vi "InitDrive.vi"   [LabVIEW 2019]
doc: "This VI initializes devices related directly to the drive subsystem."
uses:
  <vilib>/Rock Robotics/WPI/Solenoid/WPI_SolenoidChannel.ctl
  <vilib>/Rock Robotics/WPI/ThirdParty/Phoenix-LabVIEW/Motor Controller/Controls/CTRE_Phoenix_MotorControl_NeutralMode.ctl
  <vilib>/Rock Robotics/WPI/ThirdParty/Phoenix-LabVIEW/Motor Controller/Controls/CTRE_Phoenix_MotorControl_SupplyCurrentLimitConfiguration.ctl
  <vilib>/Rock Robotics/WPI/ThirdParty/Phoenix-LabVIEW/Motor Controller/Controls/CTRE_Phoenix_MotorControl_TalonFXInvertType.ctl
  <vilib>/Rock Robotics/WPI/ThirdParty/Phoenix-LabVIEW/Motor Controller/Controls/CTRE_Phoenix_MotorControl_FeedbackDevice_TalonFX.ctl
  <vilib>/Rock Robotics/WPI/Solenoid/WPI_SolenoidOpenDouble.vi
  refnums.vi
types:
  T1 = typedef "WPI_SolenoidChannel.ctl" = enum8{"Solenoid 0", "Solenoid 1", "Solenoid 2", "Solenoid 3", "Solenoid 4", "Solenoid 5", "Solenoid 6", "Solenoid 7", "Invalid"}
  T2 = typedef "CTRE_Phoenix_MotorControl_TalonFXInvertType.ctl" = enum16{"Counter-Clockwise", "Clockwise"}
  T3 = typedef "CTRE_Phoenix_MotorControl_FeedbackDevice_TalonFX.ctl" = i8
  T4 = typedef "CTRE_Phoenix_MotorControl_SupplyCurrentLimitConfiguration.ctl" = cluster{"Enable?":bool, "Current Limit":dbl, "Threshold Current":dbl, "Threshold Time":dbl}
  T5 = typedef "CTRE_Phoenix_MotorControl_NeutralMode.ctl" = enum8{"EEPROMSetting", "Override to Coast", "Override to Brake"}
  T6 = typedef "WPI_MotorControlDeviceRef.ctl" = cluster{"DeviceStatus":errorcluster, "Type":T7, "PWM":cluster{"PWM Channel":T8, "DeadBand":T9}, "CAN":cluster{"Device Number":u8, "SetOutput VI Ref":variant, "GetOutput VI Ref":variant, "Enable VI Ref":variant, "Disable VI Ref":variant, "Data":variant}, "Invert":bool, "DIO PWM":cluster{"PWM \"Enable\" Channel":T8, "DIOChannel":T10, "PWM Rate":dbl}}
  T7 = typedef "WPI_MotorControlType.ctl" = enum16{"PWM", "CAN", "DIO PWM"}
  T8 = typedef "FPGA_DIOPWMChannel.ctl" = enum8{"PWM 0", "PWM 1", "PWM 2", "PWM 3", "PWM 4", "PWM 5", "PWM 6", "PWM 7", "PWM 8", "PWM 9", "PWM MXP 0", "PWM MXP 1", "PWM MXP 2", "PWM MXP 3", "PWM MXP 4", "PWM MXP 5", "PWM MXP 6", "PWM MXP 7", "PWM MXP 8", "PWM MXP 9", "Invalid"}
  T9 = typedef "WPI_PWMDeadband.ctl" = cluster{"Name":string, "maxPositivePwm":i32, "minPositivePwm":i32, "centerPwm":i32, "maxNegativePwm":i32, "minNegativePwm":i32, "angularRange":u16}
  T10 = typedef "FPGA_DIOChannel.ctl" = enum8{"DIO 0", "DIO 1", "DIO 2", "DIO 3", "DIO 4", "DIO 5", "DIO 6", "DIO 7", "DIO 8", "DIO 9", "DIO MXP 0", "DIO MXP 1", "DIO MXP 2", "DIO MXP 3", "DIO MXP 4", "DIO MXP 5", "DIO MXP 6", "DIO MXP 7", "DIO MXP 8", "DIO MXP 9", "DIO MXP 10", "DIO MXP 11", "DIO MXP 12", "DIO MXP 13", "DIO MXP 14", "DIO MXP 15", "SPI Port CS1", "SPI Port CS2", "SPI Port CS3", "SPI Port MISO", "SPI Port MOSI", "Invalid"}
  T11 = typedef "WPI_SolenoidDevRef.ctl" = cluster{"DevStatus":errorcluster, "Pneumatics Control Module":u8, "Forward Solenoid Channel":T1, "Reverse Solenoid Channel":T1}
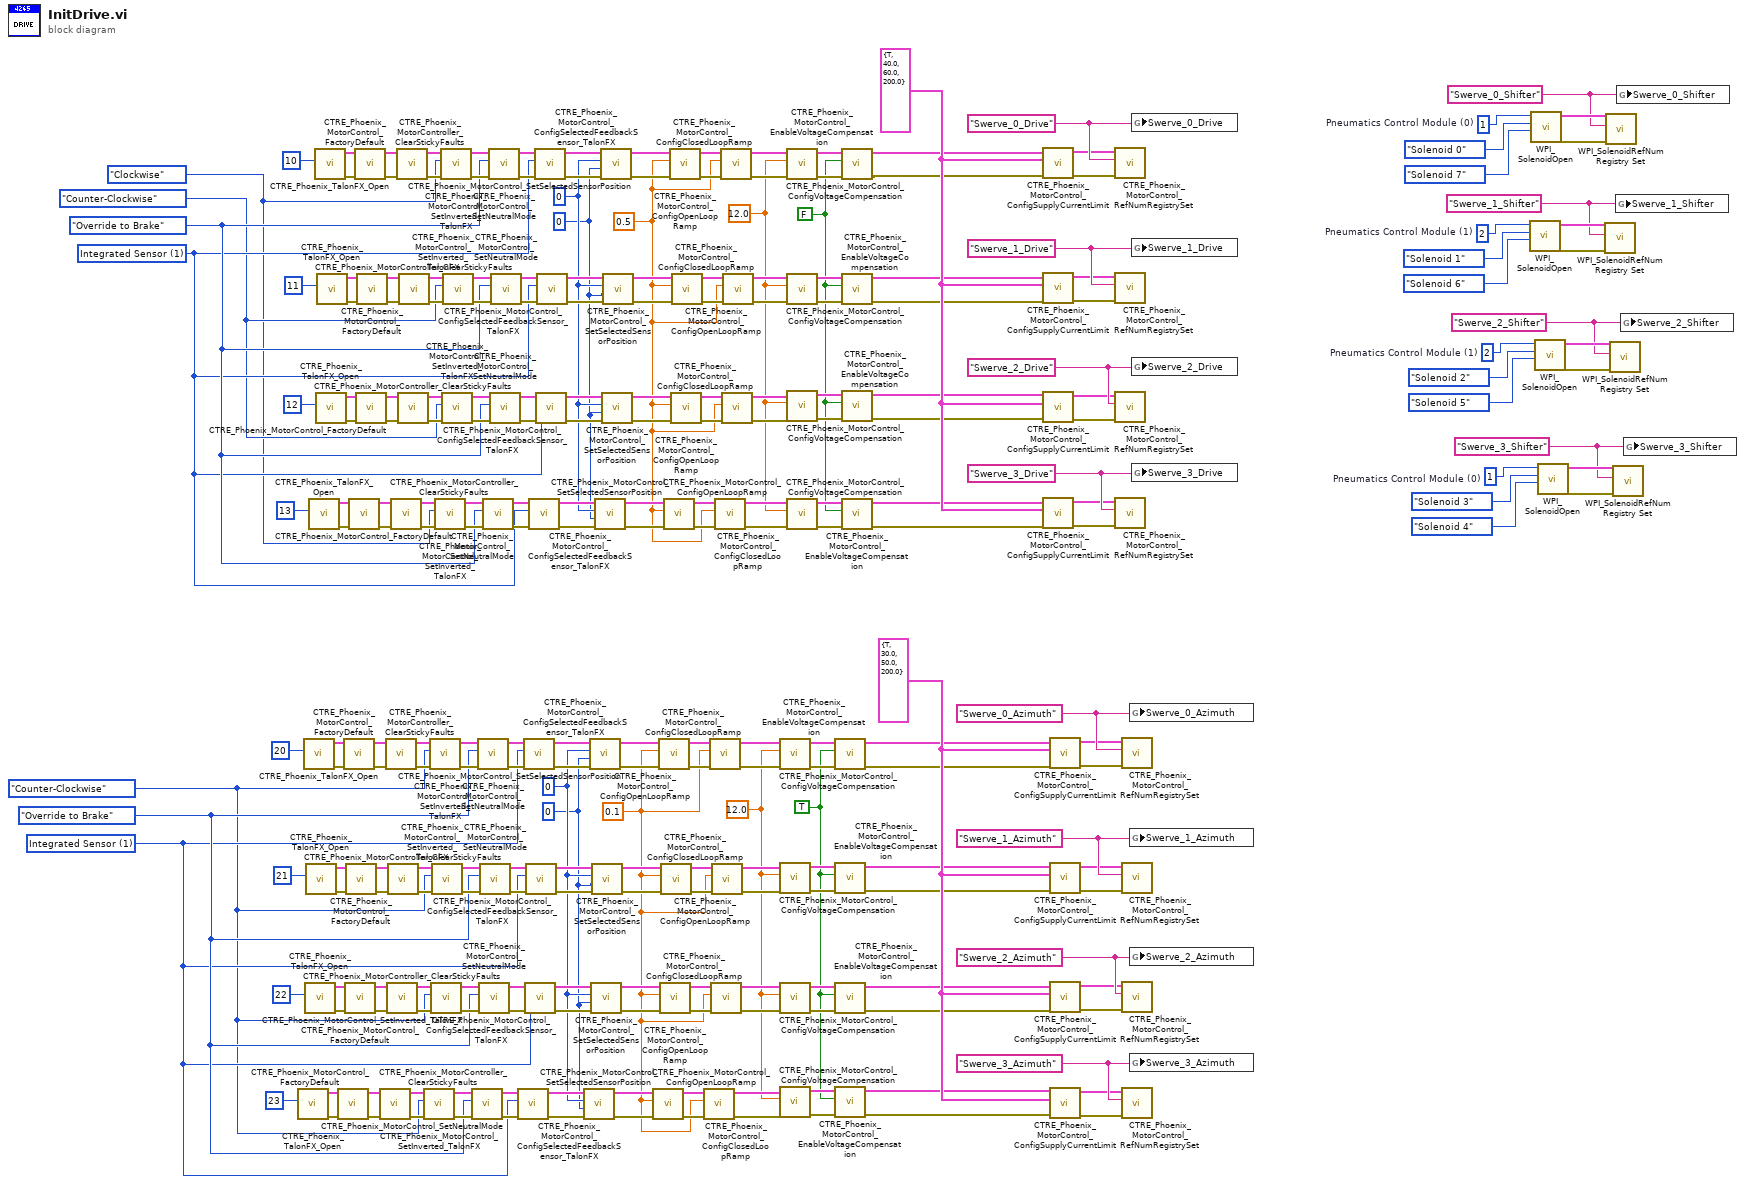
[diagram p0: block diagram]
diagram:
  w2 = "Swerve_0_Shifter" ("refnum name")
  w7 = u8 1  # Pneumatics Control Module (0)
  w8 = "Swerve_1_Shifter" ("refnum name")
  w13 = u8 2  # Pneumatics Control Module (1)
  w14 = "Swerve_2_Shifter" ("refnum name")
  w19 = u8 2  # Pneumatics Control Module (1)
  w22 = CTRE_Phoenix_MotorControl_TalonFXInvertType."Clockwise" ("Invert Type")
  w24 = TRUE ("Enable Voltage Compensation?")
  w25 = 12.0 ("Saturation Voltage")
  w26 = FALSE ("Enable Voltage Compensation?")
  w27 = 12.0 ("Saturation Voltage")
  w74 = T3 1 items=["Integrated Sensor"=1, "Sensor Sum (S0 + S1)"=9, "Sensor Difference (D0 - D1)"=10, "Remote Source 0"=11, "Remote Source 1"=12, "None"=14, "Software Emulated"=15] ("Talon FX Feedback Device")
  w79 = T4 {"Enable?"=TRUE, "Current Limit"=30.0, "Threshold Current"=50.0, "Threshold Time"=200.0} ("Supply Current Limit Configuration")
  w75 = 0.1 ("secondsFromNeutralToFull")
  w76 = u32 0 ("pidLoopIdx")
  w77 = 0 ("New Sensor Position")
  w78 = CTRE_Phoenix_MotorControl_NeutralMode."Override to Brake" ("Motor Control Neutral Mode")
  w1 = CTRE_Phoenix_MotorControl_TalonFXInvertType."Counter-Clockwise" ("Invert Type")
  w95 = "Swerve_0_Azimuth" ("refnum name")
  w115 = "Swerve_1_Azimuth" ("refnum name")
  w135 = "Swerve_2_Azimuth" ("refnum name")
  w155 = "Swerve_3_Azimuth" ("refnum name")
  w163 = T3 1 items=["Integrated Sensor"=1, "Sensor Sum (S0 + S1)"=9, "Sensor Difference (D0 - D1)"=10, "Remote Source 0"=11, "Remote Source 1"=12, "None"=14, "Software Emulated"=15] ("Talon FX Feedback Device")
  w165 = T4 {"Enable?"=TRUE, "Current Limit"=40.0, "Threshold Current"=60.0, "Threshold Time"=200.0} ("Supply Current Limit Configuration")
  w160 = 0.5 ("secondsFromNeutralToFull")
  w161 = u32 0 ("pidLoopIdx")
  w162 = 0 ("New Sensor Position")
  w164 = CTRE_Phoenix_MotorControl_NeutralMode."Override to Brake" ("Motor Control Neutral Mode")
  w23 = CTRE_Phoenix_MotorControl_TalonFXInvertType."Counter-Clockwise" ("Invert Type")
  w181 = "Swerve_0_Drive" ("refnum name")
  w201 = "Swerve_1_Drive" ("refnum name")
  w221 = "Swerve_2_Drive" ("refnum name")
  w241 = "Swerve_3_Drive" ("refnum name")
  w246 = "Swerve_3_Shifter" ("refnum name")
  w251 = u8 1  # Pneumatics Control Module (0)
  n1 = call <vilib>:"CTRE_Phoenix_TalonFX_Open.vi"("Device Number"=u8 23 ("Drive 4L")) -> ("error out"=w144:errorcluster, "CAN Talon SRX Ref"=w151:T6)  [unwired: 9 in]
  n2 = call <vilib>:"CTRE_Phoenix_TalonFX_Open.vi"("Device Number"=u8 20 ("Drive 4L")) -> ("error out"=w84:errorcluster, "CAN Talon SRX Ref"=w91:T6)  [unwired: 9 in]
  n3 = call <vilib>:"CTRE_Phoenix_TalonFX_Open.vi"("Device Number"=u8 22 ("Drive 4L")) -> ("error out"=w124:errorcluster, "CAN Talon SRX Ref"=w131:T6)  [unwired: 9 in]
  n4 = call <vilib>:"CTRE_Phoenix_TalonFX_Open.vi"("Device Number"=u8 21 ("Drive 4L")) -> ("error out"=w104:errorcluster, "CAN Talon SRX Ref"=w111:T6)  [unwired: 9 in]
  n5 = call <vilib>:"CTRE_Phoenix_TalonFX_Open.vi"("Device Number"=u8 13 ("Drive 4L")) -> ("error out"=w230:errorcluster, "CAN Talon SRX Ref"=w237:T6)  [unwired: 9 in]
  n6 = call <vilib>:"CTRE_Phoenix_TalonFX_Open.vi"("Device Number"=u8 10 ("Drive 4L")) -> ("error out"=w170:errorcluster, "CAN Talon SRX Ref"=w177:T6)  [unwired: 9 in]
  n7 = call <vilib>:"CTRE_Phoenix_TalonFX_Open.vi"("Device Number"=u8 12 ("Drive 4L")) -> ("error out"=w210:errorcluster, "CAN Talon SRX Ref"=w217:T6)  [unwired: 9 in]
  n8 = call <vilib>:"CTRE_Phoenix_TalonFX_Open.vi"("Device Number"=u8 11 ("Drive 4L")) -> ("error out"=w190:errorcluster, "CAN Talon SRX Ref"=w197:T6)  [unwired: 9 in]
  n9 = call <vilib>:"CTRE_Phoenix_MotorControl_FactoryDefault.vi"("error in"=w144, "PhoenixMotorControlDevRef"=w151) -> ("error out"=w147:errorcluster, "PhoenixMotorControlDevRef"=w148:T6)  [unwired: 8 in]
  n10 = call <vilib>:"CTRE_Phoenix_MotorControl_FactoryDefault.vi"("error in"=w84, "PhoenixMotorControlDevRef"=w91) -> ("error out"=w87:errorcluster, "PhoenixMotorControlDevRef"=w88:T6)  [unwired: 8 in]
  n11 = call <vilib>:"CTRE_Phoenix_MotorControl_FactoryDefault.vi"("error in"=w124, "PhoenixMotorControlDevRef"=w131) -> ("error out"=w127:errorcluster, "PhoenixMotorControlDevRef"=w128:T6)  [unwired: 8 in]
  n12 = call <vilib>:"CTRE_Phoenix_MotorControl_FactoryDefault.vi"("error in"=w104, "PhoenixMotorControlDevRef"=w111) -> ("error out"=w107:errorcluster, "PhoenixMotorControlDevRef"=w108:T6)  [unwired: 8 in]
  n13 = call <vilib>:"CTRE_Phoenix_MotorControl_FactoryDefault.vi"("error in"=w230, "PhoenixMotorControlDevRef"=w237) -> ("error out"=w233:errorcluster, "PhoenixMotorControlDevRef"=w234:T6)  [unwired: 8 in]
  n14 = call <vilib>:"CTRE_Phoenix_MotorControl_FactoryDefault.vi"("error in"=w170, "PhoenixMotorControlDevRef"=w177) -> ("error out"=w173:errorcluster, "PhoenixMotorControlDevRef"=w174:T6)  [unwired: 8 in]
  n15 = call <vilib>:"CTRE_Phoenix_MotorControl_FactoryDefault.vi"("error in"=w210, "PhoenixMotorControlDevRef"=w217) -> ("error out"=w213:errorcluster, "PhoenixMotorControlDevRef"=w214:T6)  [unwired: 8 in]
  n16 = call <vilib>:"CTRE_Phoenix_MotorControl_FactoryDefault.vi"("error in"=w190, "PhoenixMotorControlDevRef"=w197) -> ("error out"=w193:errorcluster, "PhoenixMotorControlDevRef"=w194:T6)  [unwired: 8 in]
  n17 = call <vilib>:"CTRE_Phoenix_MotorController_ClearStickyFaults.vi"("error in"=w147, "PhoenixMotorControlDevRef"=w148) -> ("error out"=w146:errorcluster, "PhoenixMotorControlDevRef"=w145:T6)  [unwired: 8 in]
  n18 = call <vilib>:"CTRE_Phoenix_MotorController_ClearStickyFaults.vi"("error in"=w87, "PhoenixMotorControlDevRef"=w88) -> ("error out"=w86:errorcluster, "PhoenixMotorControlDevRef"=w85:T6)  [unwired: 8 in]
  n19 = call <vilib>:"CTRE_Phoenix_MotorController_ClearStickyFaults.vi"("error in"=w127, "PhoenixMotorControlDevRef"=w128) -> ("error out"=w126:errorcluster, "PhoenixMotorControlDevRef"=w125:T6)  [unwired: 8 in]
  n20 = call <vilib>:"CTRE_Phoenix_MotorController_ClearStickyFaults.vi"("error in"=w107, "PhoenixMotorControlDevRef"=w108) -> ("error out"=w106:errorcluster, "PhoenixMotorControlDevRef"=w105:T6)  [unwired: 8 in]
  n21 = call <vilib>:"CTRE_Phoenix_MotorController_ClearStickyFaults.vi"("error in"=w233, "PhoenixMotorControlDevRef"=w234) -> ("error out"=w232:errorcluster, "PhoenixMotorControlDevRef"=w231:T6)  [unwired: 8 in]
  n22 = call <vilib>:"CTRE_Phoenix_MotorController_ClearStickyFaults.vi"("error in"=w173, "PhoenixMotorControlDevRef"=w174) -> ("error out"=w172:errorcluster, "PhoenixMotorControlDevRef"=w171:T6)  [unwired: 8 in]
  n23 = call <vilib>:"CTRE_Phoenix_MotorController_ClearStickyFaults.vi"("error in"=w213, "PhoenixMotorControlDevRef"=w214) -> ("error out"=w212:errorcluster, "PhoenixMotorControlDevRef"=w211:T6)  [unwired: 8 in]
  n24 = call <vilib>:"CTRE_Phoenix_MotorController_ClearStickyFaults.vi"("error in"=w193, "PhoenixMotorControlDevRef"=w194) -> ("error out"=w192:errorcluster, "PhoenixMotorControlDevRef"=w191:T6)  [unwired: 8 in]
  n25 = call <vilib>:"CTRE_Phoenix_MotorControl_SetInverted_TalonFX.vi"("error in (no error)"=w146, "Invert Type"=w1, "PhoenixMotorControlDevRef"=w145) -> ("error out"=w158:errorcluster, "PhoenixMotorControlDevRef"=w159:T6)  [unwired: 7 in]
  n26 = call <vilib>:"CTRE_Phoenix_MotorControl_SetInverted_TalonFX.vi"("error in (no error)"=w86, "Invert Type"=w1, "PhoenixMotorControlDevRef"=w85) -> ("error out"=w98:errorcluster, "PhoenixMotorControlDevRef"=w99:T6)  [unwired: 7 in]
  n27 = call <vilib>:"CTRE_Phoenix_MotorControl_SetInverted_TalonFX.vi"("error in (no error)"=w126, "Invert Type"=w1, "PhoenixMotorControlDevRef"=w125) -> ("error out"=w138:errorcluster, "PhoenixMotorControlDevRef"=w139:T6)  [unwired: 7 in]
  n28 = call <vilib>:"CTRE_Phoenix_MotorControl_SetInverted_TalonFX.vi"("error in (no error)"=w106, "Invert Type"=w1, "PhoenixMotorControlDevRef"=w105) -> ("error out"=w118:errorcluster, "PhoenixMotorControlDevRef"=w119:T6)  [unwired: 7 in]
  n29 = call <vilib>:"CTRE_Phoenix_MotorControl_SetInverted_TalonFX.vi"("error in (no error)"=w232, "Invert Type"=w22, "PhoenixMotorControlDevRef"=w231) -> ("error out"=w244:errorcluster, "PhoenixMotorControlDevRef"=w245:T6)  [unwired: 7 in]
  n30 = call <vilib>:"CTRE_Phoenix_MotorControl_SetInverted_TalonFX.vi"("error in (no error)"=w172, "Invert Type"=w22, "PhoenixMotorControlDevRef"=w171) -> ("error out"=w184:errorcluster, "PhoenixMotorControlDevRef"=w185:T6)  [unwired: 7 in]
  n31 = call <vilib>:"CTRE_Phoenix_MotorControl_SetInverted_TalonFX.vi"("error in (no error)"=w212, "Invert Type"=w23, "PhoenixMotorControlDevRef"=w211) -> ("error out"=w224:errorcluster, "PhoenixMotorControlDevRef"=w225:T6)  [unwired: 7 in]
  n32 = call <vilib>:"CTRE_Phoenix_MotorControl_SetInverted_TalonFX.vi"("error in (no error)"=w192, "Invert Type"=w23, "PhoenixMotorControlDevRef"=w191) -> ("error out"=w204:errorcluster, "PhoenixMotorControlDevRef"=w205:T6)  [unwired: 7 in]
  n33 = call <vilib>:"CTRE_Phoenix_MotorControl_SetNeutralMode.vi"("error in (no error)"=w158, "Motor Control Neutral Mode"=w78, "PhoenixMotorControlDevRef"=w159) -> ("error out"=w142:errorcluster, "PhoenixMotorControlDevRef"=w143:T6)  [unwired: 7 in]
  n34 = call <vilib>:"CTRE_Phoenix_MotorControl_SetNeutralMode.vi"("error in (no error)"=w98, "Motor Control Neutral Mode"=w78, "PhoenixMotorControlDevRef"=w99) -> ("error out"=w82:errorcluster, "PhoenixMotorControlDevRef"=w83:T6)  [unwired: 7 in]
  n35 = call <vilib>:"CTRE_Phoenix_MotorControl_SetNeutralMode.vi"("error in (no error)"=w138, "Motor Control Neutral Mode"=w78, "PhoenixMotorControlDevRef"=w139) -> ("error out"=w122:errorcluster, "PhoenixMotorControlDevRef"=w123:T6)  [unwired: 7 in]
  n36 = call <vilib>:"CTRE_Phoenix_MotorControl_SetNeutralMode.vi"("error in (no error)"=w118, "Motor Control Neutral Mode"=w78, "PhoenixMotorControlDevRef"=w119) -> ("error out"=w102:errorcluster, "PhoenixMotorControlDevRef"=w103:T6)  [unwired: 7 in]
  n37 = call <vilib>:"CTRE_Phoenix_MotorControl_SetNeutralMode.vi"("error in (no error)"=w244, "Motor Control Neutral Mode"=w164, "PhoenixMotorControlDevRef"=w245) -> ("error out"=w228:errorcluster, "PhoenixMotorControlDevRef"=w229:T6)  [unwired: 7 in]
  n38 = call <vilib>:"CTRE_Phoenix_MotorControl_SetNeutralMode.vi"("error in (no error)"=w184, "Motor Control Neutral Mode"=w164, "PhoenixMotorControlDevRef"=w185) -> ("error out"=w168:errorcluster, "PhoenixMotorControlDevRef"=w169:T6)  [unwired: 7 in]
  n39 = call <vilib>:"CTRE_Phoenix_MotorControl_SetNeutralMode.vi"("error in (no error)"=w224, "Motor Control Neutral Mode"=w164, "PhoenixMotorControlDevRef"=w225) -> ("error out"=w208:errorcluster, "PhoenixMotorControlDevRef"=w209:T6)  [unwired: 7 in]
  n40 = call <vilib>:"CTRE_Phoenix_MotorControl_SetNeutralMode.vi"("error in (no error)"=w204, "Motor Control Neutral Mode"=w164, "PhoenixMotorControlDevRef"=w205) -> ("error out"=w188:errorcluster, "PhoenixMotorControlDevRef"=w189:T6)  [unwired: 7 in]
  n41 = call <vilib>:"CTRE_Phoenix_MotorControl_ConfigSelectedFeedbackSensor_TalonFX.vi"("error in (no error)"=w142, "Talon FX Feedback Device"=w74, "PhoenixMotorControlDevRef"=w143) -> ("error out"=w140:errorcluster, "PhoenixMotorControlDevRef"=w141:T6)  [unwired: 7 in]
  n42 = call <vilib>:"CTRE_Phoenix_MotorControl_ConfigSelectedFeedbackSensor_TalonFX.vi"("error in (no error)"=w82, "Talon FX Feedback Device"=w74, "PhoenixMotorControlDevRef"=w83) -> ("error out"=w80:errorcluster, "PhoenixMotorControlDevRef"=w81:T6)  [unwired: 7 in]
  n43 = call <vilib>:"CTRE_Phoenix_MotorControl_ConfigSelectedFeedbackSensor_TalonFX.vi"("error in (no error)"=w122, "Talon FX Feedback Device"=w74, "PhoenixMotorControlDevRef"=w123) -> ("error out"=w120:errorcluster, "PhoenixMotorControlDevRef"=w121:T6)  [unwired: 7 in]
  n44 = call <vilib>:"CTRE_Phoenix_MotorControl_ConfigSelectedFeedbackSensor_TalonFX.vi"("error in (no error)"=w102, "Talon FX Feedback Device"=w74, "PhoenixMotorControlDevRef"=w103) -> ("error out"=w100:errorcluster, "PhoenixMotorControlDevRef"=w101:T6)  [unwired: 7 in]
  n45 = call <vilib>:"CTRE_Phoenix_MotorControl_ConfigSelectedFeedbackSensor_TalonFX.vi"("error in (no error)"=w228, "Talon FX Feedback Device"=w163, "PhoenixMotorControlDevRef"=w229) -> ("error out"=w226:errorcluster, "PhoenixMotorControlDevRef"=w227:T6)  [unwired: 7 in]
  n46 = call <vilib>:"CTRE_Phoenix_MotorControl_ConfigSelectedFeedbackSensor_TalonFX.vi"("error in (no error)"=w168, "Talon FX Feedback Device"=w163, "PhoenixMotorControlDevRef"=w169) -> ("error out"=w166:errorcluster, "PhoenixMotorControlDevRef"=w167:T6)  [unwired: 7 in]
  n47 = call <vilib>:"CTRE_Phoenix_MotorControl_ConfigSelectedFeedbackSensor_TalonFX.vi"("error in (no error)"=w208, "Talon FX Feedback Device"=w163, "PhoenixMotorControlDevRef"=w209) -> ("error out"=w206:errorcluster, "PhoenixMotorControlDevRef"=w207:T6)  [unwired: 7 in]
  n48 = call <vilib>:"CTRE_Phoenix_MotorControl_ConfigSelectedFeedbackSensor_TalonFX.vi"("error in (no error)"=w188, "Talon FX Feedback Device"=w163, "PhoenixMotorControlDevRef"=w189) -> ("error out"=w186:errorcluster, "PhoenixMotorControlDevRef"=w187:T6)  [unwired: 7 in]
  n49 = call <vilib>:"CTRE_Phoenix_MotorControl_SetSelectedSensorPosition.vi"("error in (no error)"=w140, "pidLoopIdx"=w76, "New Sensor Position"=w77, "PhoenixMotorControlDevRef"=w141) -> ("error out"=w157:errorcluster, "PhoenixMotorControlDevRef"=w156:T6)  [unwired: 6 in]
  n50 = call <vilib>:"CTRE_Phoenix_MotorControl_SetSelectedSensorPosition.vi"("error in (no error)"=w80, "pidLoopIdx"=w76, "New Sensor Position"=w77, "PhoenixMotorControlDevRef"=w81) -> ("error out"=w97:errorcluster, "PhoenixMotorControlDevRef"=w96:T6)  [unwired: 6 in]
  n51 = call <vilib>:"CTRE_Phoenix_MotorControl_SetSelectedSensorPosition.vi"("error in (no error)"=w120, "pidLoopIdx"=w76, "New Sensor Position"=w77, "PhoenixMotorControlDevRef"=w121) -> ("error out"=w137:errorcluster, "PhoenixMotorControlDevRef"=w136:T6)  [unwired: 6 in]
  n52 = call <vilib>:"CTRE_Phoenix_MotorControl_SetSelectedSensorPosition.vi"("error in (no error)"=w100, "pidLoopIdx"=w76, "New Sensor Position"=w77, "PhoenixMotorControlDevRef"=w101) -> ("error out"=w117:errorcluster, "PhoenixMotorControlDevRef"=w116:T6)  [unwired: 6 in]
  n53 = call <vilib>:"CTRE_Phoenix_MotorControl_SetSelectedSensorPosition.vi"("error in (no error)"=w226, "pidLoopIdx"=w161, "New Sensor Position"=w162, "PhoenixMotorControlDevRef"=w227) -> ("error out"=w243:errorcluster, "PhoenixMotorControlDevRef"=w242:T6)  [unwired: 6 in]
  n54 = call <vilib>:"CTRE_Phoenix_MotorControl_SetSelectedSensorPosition.vi"("error in (no error)"=w166, "pidLoopIdx"=w161, "New Sensor Position"=w162, "PhoenixMotorControlDevRef"=w167) -> ("error out"=w183:errorcluster, "PhoenixMotorControlDevRef"=w182:T6)  [unwired: 6 in]
  n55 = call <vilib>:"CTRE_Phoenix_MotorControl_SetSelectedSensorPosition.vi"("error in (no error)"=w206, "pidLoopIdx"=w161, "New Sensor Position"=w162, "PhoenixMotorControlDevRef"=w207) -> ("error out"=w223:errorcluster, "PhoenixMotorControlDevRef"=w222:T6)  [unwired: 6 in]
  n56 = call <vilib>:"CTRE_Phoenix_MotorControl_SetSelectedSensorPosition.vi"("error in (no error)"=w186, "pidLoopIdx"=w161, "New Sensor Position"=w162, "PhoenixMotorControlDevRef"=w187) -> ("error out"=w203:errorcluster, "PhoenixMotorControlDevRef"=w202:T6)  [unwired: 6 in]
  n57 = call <vilib>:"CTRE_Phoenix_MotorControl_ConfigOpenLoopRamp.vi"("error in (no error)"=w157, "secondsFromNeutralToFull"=w75, "PhoenixMotorControlDevRef"=w156) -> ("error out"=w149:errorcluster, "PhoenixMotorControlDevRef"=w150:T6)  [unwired: 7 in]
  n58 = call <vilib>:"CTRE_Phoenix_MotorControl_ConfigOpenLoopRamp.vi"("error in (no error)"=w97, "secondsFromNeutralToFull"=w75, "PhoenixMotorControlDevRef"=w96) -> ("error out"=w89:errorcluster, "PhoenixMotorControlDevRef"=w90:T6)  [unwired: 7 in]
  n59 = call <vilib>:"CTRE_Phoenix_MotorControl_ConfigOpenLoopRamp.vi"("error in (no error)"=w137, "secondsFromNeutralToFull"=w75, "PhoenixMotorControlDevRef"=w136) -> ("error out"=w129:errorcluster, "PhoenixMotorControlDevRef"=w130:T6)  [unwired: 7 in]
  n60 = call <vilib>:"CTRE_Phoenix_MotorControl_ConfigOpenLoopRamp.vi"("error in (no error)"=w117, "secondsFromNeutralToFull"=w75, "PhoenixMotorControlDevRef"=w116) -> ("error out"=w109:errorcluster, "PhoenixMotorControlDevRef"=w110:T6)  [unwired: 7 in]
  n61 = call <vilib>:"CTRE_Phoenix_MotorControl_ConfigOpenLoopRamp.vi"("error in (no error)"=w243, "secondsFromNeutralToFull"=w160, "PhoenixMotorControlDevRef"=w242) -> ("error out"=w235:errorcluster, "PhoenixMotorControlDevRef"=w236:T6)  [unwired: 7 in]
  n62 = call <vilib>:"CTRE_Phoenix_MotorControl_ConfigOpenLoopRamp.vi"("error in (no error)"=w183, "secondsFromNeutralToFull"=w160, "PhoenixMotorControlDevRef"=w182) -> ("error out"=w175:errorcluster, "PhoenixMotorControlDevRef"=w176:T6)  [unwired: 7 in]
  n63 = call <vilib>:"CTRE_Phoenix_MotorControl_ConfigOpenLoopRamp.vi"("error in (no error)"=w223, "secondsFromNeutralToFull"=w160, "PhoenixMotorControlDevRef"=w222) -> ("error out"=w215:errorcluster, "PhoenixMotorControlDevRef"=w216:T6)  [unwired: 7 in]
  n64 = call <vilib>:"CTRE_Phoenix_MotorControl_ConfigOpenLoopRamp.vi"("error in (no error)"=w203, "secondsFromNeutralToFull"=w160, "PhoenixMotorControlDevRef"=w202) -> ("error out"=w195:errorcluster, "PhoenixMotorControlDevRef"=w196:T6)  [unwired: 7 in]
  n65 = call <vilib>:"CTRE_Phoenix_MotorControl_ConfigClosedLoopRamp.vi"("error in (no error)"=w149, "secondsFromNeutralToFull"=w75, "PhoenixMotorControlDevRef"=w150) -> ("error out"=w30:errorcluster, "PhoenixMotorControlDevRef"=w31:T6)  [unwired: 7 in]
  n66 = call <vilib>:"CTRE_Phoenix_MotorControl_ConfigClosedLoopRamp.vi"("error in (no error)"=w89, "secondsFromNeutralToFull"=w75, "PhoenixMotorControlDevRef"=w90) -> ("error out"=w42:errorcluster, "PhoenixMotorControlDevRef"=w43:T6)  [unwired: 7 in]
  n67 = call <vilib>:"CTRE_Phoenix_MotorControl_ConfigClosedLoopRamp.vi"("error in (no error)"=w129, "secondsFromNeutralToFull"=w75, "PhoenixMotorControlDevRef"=w130) -> ("error out"=w34:errorcluster, "PhoenixMotorControlDevRef"=w35:T6)  [unwired: 7 in]
  n68 = call <vilib>:"CTRE_Phoenix_MotorControl_ConfigClosedLoopRamp.vi"("error in (no error)"=w109, "secondsFromNeutralToFull"=w75, "PhoenixMotorControlDevRef"=w110) -> ("error out"=w38:errorcluster, "PhoenixMotorControlDevRef"=w39:T6)  [unwired: 7 in]
  n69 = call <vilib>:"CTRE_Phoenix_MotorControl_ConfigClosedLoopRamp.vi"("error in (no error)"=w235, "secondsFromNeutralToFull"=w160, "PhoenixMotorControlDevRef"=w236) -> ("error out"=w46:errorcluster, "PhoenixMotorControlDevRef"=w47:T6)  [unwired: 7 in]
  n70 = call <vilib>:"CTRE_Phoenix_MotorControl_ConfigClosedLoopRamp.vi"("error in (no error)"=w175, "secondsFromNeutralToFull"=w160, "PhoenixMotorControlDevRef"=w176) -> ("error out"=w56:errorcluster, "PhoenixMotorControlDevRef"=w57:T6)  [unwired: 7 in]
  n71 = call <vilib>:"CTRE_Phoenix_MotorControl_ConfigClosedLoopRamp.vi"("error in (no error)"=w215, "secondsFromNeutralToFull"=w160, "PhoenixMotorControlDevRef"=w216) -> ("error out"=w50:errorcluster, "PhoenixMotorControlDevRef"=w51:T6)  [unwired: 7 in]
  n72 = call <vilib>:"CTRE_Phoenix_MotorControl_ConfigClosedLoopRamp.vi"("error in (no error)"=w195, "secondsFromNeutralToFull"=w160, "PhoenixMotorControlDevRef"=w196) -> ("error out"=w54:errorcluster, "PhoenixMotorControlDevRef"=w55:T6)  [unwired: 7 in]
  n73 = call <vilib>:"CTRE_Phoenix_MotorControl_ConfigVoltageCompensation.vi"("error in (no error)"=w42, "Saturation Voltage"=w25, "PhoenixMotorControlDevRef"=w43) -> ("error out"=w64:errorcluster, "PhoenixMotorControlDevRef"=w65:T6)  [unwired: 7 in]
  n74 = call <vilib>:"CTRE_Phoenix_MotorControl_ConfigVoltageCompensation.vi"("error in (no error)"=w38, "Saturation Voltage"=w25, "PhoenixMotorControlDevRef"=w39) -> ("error out"=w62:errorcluster, "PhoenixMotorControlDevRef"=w63:T6)  [unwired: 7 in]
  n75 = call <vilib>:"CTRE_Phoenix_MotorControl_ConfigVoltageCompensation.vi"("error in (no error)"=w34, "Saturation Voltage"=w25, "PhoenixMotorControlDevRef"=w35) -> ("error out"=w60:errorcluster, "PhoenixMotorControlDevRef"=w61:T6)  [unwired: 7 in]
  n76 = call <vilib>:"CTRE_Phoenix_MotorControl_ConfigVoltageCompensation.vi"("error in (no error)"=w30, "Saturation Voltage"=w25, "PhoenixMotorControlDevRef"=w31) -> ("error out"=w58:errorcluster, "PhoenixMotorControlDevRef"=w59:T6)  [unwired: 7 in]
  n77 = call <vilib>:"CTRE_Phoenix_MotorControl_ConfigVoltageCompensation.vi"("error in (no error)"=w56, "Saturation Voltage"=w27, "PhoenixMotorControlDevRef"=w57) -> ("error out"=w72:errorcluster, "PhoenixMotorControlDevRef"=w73:T6)  [unwired: 7 in]
  n78 = call <vilib>:"CTRE_Phoenix_MotorControl_ConfigVoltageCompensation.vi"("error in (no error)"=w54, "Saturation Voltage"=w27, "PhoenixMotorControlDevRef"=w55) -> ("error out"=w70:errorcluster, "PhoenixMotorControlDevRef"=w71:T6)  [unwired: 7 in]
  n79 = call <vilib>:"CTRE_Phoenix_MotorControl_ConfigVoltageCompensation.vi"("error in (no error)"=w50, "Saturation Voltage"=w27, "PhoenixMotorControlDevRef"=w51) -> ("error out"=w68:errorcluster, "PhoenixMotorControlDevRef"=w69:T6)  [unwired: 7 in]
  n80 = call <vilib>:"CTRE_Phoenix_MotorControl_ConfigVoltageCompensation.vi"("error in (no error)"=w46, "Saturation Voltage"=w27, "PhoenixMotorControlDevRef"=w47) -> ("error out"=w66:errorcluster, "PhoenixMotorControlDevRef"=w67:T6)  [unwired: 7 in]
  n81 = call <vilib>:"CTRE_Phoenix_MotorControl_EnableVoltageCompensation.vi"("error in (no error)"=w64, "Enable Voltage Compensation?"=w24, "PhoenixMotorControlDevRef"=w65) -> ("error out"=w40:errorcluster, "PhoenixMotorControlDevRef"=w41:T6)  [unwired: 7 in]
  n82 = call <vilib>:"CTRE_Phoenix_MotorControl_EnableVoltageCompensation.vi"("error in (no error)"=w62, "Enable Voltage Compensation?"=w24, "PhoenixMotorControlDevRef"=w63) -> ("error out"=w36:errorcluster, "PhoenixMotorControlDevRef"=w37:T6)  [unwired: 7 in]
  n83 = call <vilib>:"CTRE_Phoenix_MotorControl_EnableVoltageCompensation.vi"("error in (no error)"=w60, "Enable Voltage Compensation?"=w24, "PhoenixMotorControlDevRef"=w61) -> ("error out"=w32:errorcluster, "PhoenixMotorControlDevRef"=w33:T6)  [unwired: 7 in]
  n84 = call <vilib>:"CTRE_Phoenix_MotorControl_EnableVoltageCompensation.vi"("error in (no error)"=w58, "Enable Voltage Compensation?"=w24, "PhoenixMotorControlDevRef"=w59) -> ("error out"=w28:errorcluster, "PhoenixMotorControlDevRef"=w29:T6)  [unwired: 7 in]
  n85 = call <vilib>:"CTRE_Phoenix_MotorControl_EnableVoltageCompensation.vi"("error in (no error)"=w72, "Enable Voltage Compensation?"=w26, "PhoenixMotorControlDevRef"=w73) -> ("error out"=w20:errorcluster, "PhoenixMotorControlDevRef"=w21:T6)  [unwired: 7 in]
  n86 = call <vilib>:"CTRE_Phoenix_MotorControl_EnableVoltageCompensation.vi"("error in (no error)"=w70, "Enable Voltage Compensation?"=w26, "PhoenixMotorControlDevRef"=w71) -> ("error out"=w52:errorcluster, "PhoenixMotorControlDevRef"=w53:T6)  [unwired: 7 in]
  n87 = call <vilib>:"CTRE_Phoenix_MotorControl_EnableVoltageCompensation.vi"("error in (no error)"=w68, "Enable Voltage Compensation?"=w26, "PhoenixMotorControlDevRef"=w69) -> ("error out"=w48:errorcluster, "PhoenixMotorControlDevRef"=w49:T6)  [unwired: 7 in]
  n88 = call <vilib>:"CTRE_Phoenix_MotorControl_EnableVoltageCompensation.vi"("error in (no error)"=w66, "Enable Voltage Compensation?"=w26, "PhoenixMotorControlDevRef"=w67) -> ("error out"=w44:errorcluster, "PhoenixMotorControlDevRef"=w45:T6)  [unwired: 7 in]
  n89 = call <vilib>:"CTRE_Phoenix_MotorControl_ConfigSupplyCurrentLimit.vi"("error in (no error)"=w20, "Supply Current Limit Configuration"=w165, "PhoenixMotorControlDevRef"=w21) -> ("error out"=w179:errorcluster, "PhoenixMotorControlDevRef"=w180:T6)  [unwired: 7 in]
  n90 = call <vilib>:"CTRE_Phoenix_MotorControl_ConfigSupplyCurrentLimit.vi"("error in (no error)"=w52, "Supply Current Limit Configuration"=w165, "PhoenixMotorControlDevRef"=w53) -> ("error out"=w199:errorcluster, "PhoenixMotorControlDevRef"=w200:T6)  [unwired: 7 in]
  n91 = call <vilib>:"CTRE_Phoenix_MotorControl_ConfigSupplyCurrentLimit.vi"("error in (no error)"=w48, "Supply Current Limit Configuration"=w165, "PhoenixMotorControlDevRef"=w49) -> ("error out"=w219:errorcluster, "PhoenixMotorControlDevRef"=w220:T6)  [unwired: 7 in]
  n92 = call <vilib>:"CTRE_Phoenix_MotorControl_ConfigSupplyCurrentLimit.vi"("error in (no error)"=w44, "Supply Current Limit Configuration"=w165, "PhoenixMotorControlDevRef"=w45) -> ("error out"=w239:errorcluster, "PhoenixMotorControlDevRef"=w240:T6)  [unwired: 7 in]
  n93 = call <vilib>:"CTRE_Phoenix_MotorControl_ConfigSupplyCurrentLimit.vi"("error in (no error)"=w40, "Supply Current Limit Configuration"=w79, "PhoenixMotorControlDevRef"=w41) -> ("error out"=w93:errorcluster, "PhoenixMotorControlDevRef"=w94:T6)  [unwired: 7 in]
  n94 = call <vilib>:"CTRE_Phoenix_MotorControl_ConfigSupplyCurrentLimit.vi"("error in (no error)"=w36, "Supply Current Limit Configuration"=w79, "PhoenixMotorControlDevRef"=w37) -> ("error out"=w113:errorcluster, "PhoenixMotorControlDevRef"=w114:T6)  [unwired: 7 in]
  n95 = call <vilib>:"CTRE_Phoenix_MotorControl_ConfigSupplyCurrentLimit.vi"("error in (no error)"=w32, "Supply Current Limit Configuration"=w79, "PhoenixMotorControlDevRef"=w33) -> ("error out"=w133:errorcluster, "PhoenixMotorControlDevRef"=w134:T6)  [unwired: 7 in]
  n96 = call <vilib>:"CTRE_Phoenix_MotorControl_ConfigSupplyCurrentLimit.vi"("error in (no error)"=w28, "Supply Current Limit Configuration"=w79, "PhoenixMotorControlDevRef"=w29) -> ("error out"=w153:errorcluster, "PhoenixMotorControlDevRef"=w154:T6)  [unwired: 7 in]
  n97 = call <vilib>:"CTRE_Phoenix_MotorControl_RefNumRegistrySet.vi"("error in (no error)"=w179, "refnum name"=w181, "PhoenixMotorControlDevRef"=w180) -> ()  [unwired: 7 in, 2 out]
  n98 = call <vilib>:"CTRE_Phoenix_MotorControl_RefNumRegistrySet.vi"("error in (no error)"=w199, "refnum name"=w201, "PhoenixMotorControlDevRef"=w200) -> ()  [unwired: 7 in, 2 out]
  n99 = call <vilib>:"CTRE_Phoenix_MotorControl_RefNumRegistrySet.vi"("error in (no error)"=w219, "refnum name"=w221, "PhoenixMotorControlDevRef"=w220) -> ()  [unwired: 7 in, 2 out]
  n100 = call <vilib>:"CTRE_Phoenix_MotorControl_RefNumRegistrySet.vi"("error in (no error)"=w239, "refnum name"=w241, "PhoenixMotorControlDevRef"=w240) -> ()  [unwired: 7 in, 2 out]
  n101 = call <vilib>:"CTRE_Phoenix_MotorControl_RefNumRegistrySet.vi"("error in (no error)"=w93, "refnum name"=w95, "PhoenixMotorControlDevRef"=w94) -> ()  [unwired: 7 in, 2 out]
  n102 = call <vilib>:"CTRE_Phoenix_MotorControl_RefNumRegistrySet.vi"("error in (no error)"=w113, "refnum name"=w115, "PhoenixMotorControlDevRef"=w114) -> ()  [unwired: 7 in, 2 out]
  n103 = call <vilib>:"CTRE_Phoenix_MotorControl_RefNumRegistrySet.vi"("error in (no error)"=w133, "refnum name"=w135, "PhoenixMotorControlDevRef"=w134) -> ()  [unwired: 7 in, 2 out]
  n104 = call <vilib>:"CTRE_Phoenix_MotorControl_RefNumRegistrySet.vi"("error in (no error)"=w153, "refnum name"=w155, "PhoenixMotorControlDevRef"=w154) -> ()  [unwired: 7 in, 2 out]
  n105 = global write "refnums.vi" "Swerve_0_Azimuth"(w95) -> ()
  n106 = global write "refnums.vi" "Swerve_1_Azimuth"(w115) -> ()
  n107 = global write "refnums.vi" "Swerve_2_Azimuth"(w135) -> ()
  n108 = global write "refnums.vi" "Swerve_3_Azimuth"(w155) -> ()
  n109 = global write "refnums.vi" "Swerve_0_Drive"(w181) -> ()
  n110 = global write "refnums.vi" "Swerve_1_Drive"(w201) -> ()
  n111 = global write "refnums.vi" "Swerve_2_Drive"(w221) -> ()
  n112 = global write "refnums.vi" "Swerve_3_Drive"(w241) -> ()
  n113 = call-poly <vilib>:"WPI_SolenoidOpen.vi"("Reverse Solenoid Channel"=WPI_SolenoidChannel."Solenoid 6", "Forward Solenoid Channel"=WPI_SolenoidChannel."Solenoid 1", "Pneumatics Control Module (0)"=w13) -> ("error out"=w9:errorcluster, "SolenoidDevRef"=w10:T11)  [unwired: 7 in]
  n114 = call-poly <vilib>:"WPI_SolenoidOpen.vi"("Reverse Solenoid Channel"=WPI_SolenoidChannel."Solenoid 7", "Forward Solenoid Channel"=WPI_SolenoidChannel."Solenoid 0", "Pneumatics Control Module (0)"=w7) -> ("error out"=w3:errorcluster, "SolenoidDevRef"=w4:T11)  [unwired: 7 in]
  n115 = call-poly <vilib>:"WPI_SolenoidOpen.vi"("Reverse Solenoid Channel"=WPI_SolenoidChannel."Solenoid 5", "Forward Solenoid Channel"=WPI_SolenoidChannel."Solenoid 2", "Pneumatics Control Module (0)"=w19) -> ("error out"=w15:errorcluster, "SolenoidDevRef"=w16:T11)  [unwired: 7 in]
  n116 = call-poly <vilib>:"WPI_SolenoidOpen.vi"("Reverse Solenoid Channel"=WPI_SolenoidChannel."Solenoid 4", "Forward Solenoid Channel"=WPI_SolenoidChannel."Solenoid 3", "Pneumatics Control Module (0)"=w251) -> ("error out"=w247:errorcluster, "SolenoidDevRef"=w248:T11)  [unwired: 7 in]
  n117 = call <vilib>:"WPI_SolenoidRefNum Registry Set.vi"("error in (no error)"=w9, "refnum name"=w8, "SolenoidDevRef"=w10) -> ()  [unwired: 7 in, 2 out]
  n118 = call <vilib>:"WPI_SolenoidRefNum Registry Set.vi"("error in (no error)"=w3, "refnum name"=w2, "SolenoidDevRef"=w4) -> ()  [unwired: 7 in, 2 out]
  n119 = call <vilib>:"WPI_SolenoidRefNum Registry Set.vi"("error in (no error)"=w15, "refnum name"=w14, "SolenoidDevRef"=w16) -> ()  [unwired: 7 in, 2 out]
  n120 = call <vilib>:"WPI_SolenoidRefNum Registry Set.vi"("error in (no error)"=w247, "refnum name"=w246, "SolenoidDevRef"=w248) -> ()  [unwired: 7 in, 2 out]
  n121 = global write "refnums.vi" "Swerve_1_Shifter"(w8) -> ()
  n122 = global write "refnums.vi" "Swerve_0_Shifter"(w2) -> ()
  n123 = global write "refnums.vi" "Swerve_2_Shifter"(w14) -> ()
  n124 = global write "refnums.vi" "Swerve_3_Shifter"(w246) -> ()
